vi "Read RP Modulated Configuration.vi"(8 "error in (no error)":errorcluster, 11 "Red Pitaya Modulated Digitizer in":refnum<class "Red Pitaya Modulated Digitizer.lvclass">) -> (0 "error out":errorcluster, 2 "Configuration":T1={"Pre-trigger duration"=0.01, "Post-trigger duration"=0.1, "Rate"=125000000.0, "Ranges"=[1.0], "Re-name channels"=[], "Active channels"="0:1", "External clock"=FALSE, "Modulation"={"Output delay"=0.001, "After delay"=FALSE}} {"Modulation"."Output delay" format="%#_6ps"; "Rate" format="%#_8pHz"; "Post-trigger duration" format="%#_6ps"; "Pre-trigger duration" format="%#_6ps"; "Ranges" format="%#_6pV"}, 3 "Red Pitaya Modulated Digitizer out":refnum<class "Red Pitaya Modulated Digitizer.lvclass">)   [LabVIEW 2020, in "Red Pitaya Modulated Digitizer.lvclass"]
uses:
  Red Pitaya Modulated Digitizer.lvclass
  C:/GitHub/NHMFL_Core/Libraries/Instruments/Instrument Driver/Instrument Driver.lvclass
  RP Modulated Configuration.ctl
  Modulation.ctl
  Instruments/Instrument Driver/Read User configuration.vi
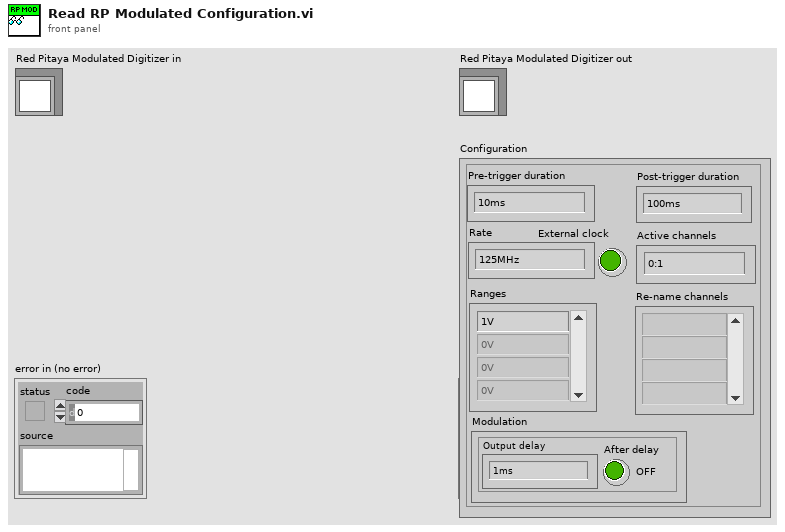
[diagram p1: front panel]
types:
  T1 = typedef "RP Modulated Configuration.ctl" = cluster{"Pre-trigger duration":dbl, "Post-trigger duration":dbl, "Rate":dbl, "Ranges":dbl[], "Re-name channels":string[], "Active channels":string, "External clock":bool, "Modulation":T2}
  T2 = typedef "Modulation.ctl" = cluster{"Output delay":dbl, "After delay":bool}
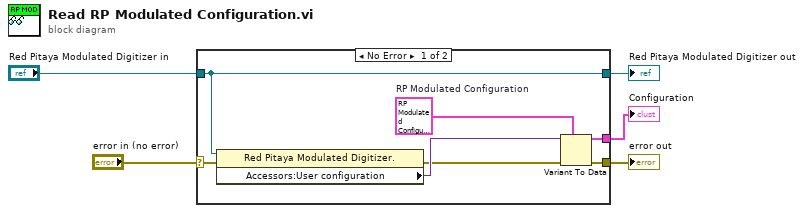
[diagram p0: block diagram]
diagram:
  n1 = case shown="No Error" "error in (no error)" {
    selector: "error in (no error)" -> [w10 w13]
    tunnel: [w8 w13] -> w4
    tunnel: [w11 w14] -> w2
    tunnel: "Red Pitaya Modulated Digitizer in" -> [w11 w14]
    tunnel: [w6 _] -> w1
    frame No Error {
      w7 = T1 {"Pre-trigger duration"=0.01, "Post-trigger duration"=0.1, "Rate"=125000000.0, "Ranges"=[1.0], "Re-name channels"=[], "Active channels"="0:1", "External clock"=FALSE, "Modulation"={"Output delay"=0.001, "After delay"=FALSE}}  # RP Modulated Configuration
      n2 = property class="Red Pitaya Modulated Digitizer."(reference=w11, error in=w10) -> (error out=w9:errorcluster, "Accessors:User configuration"=w12:variant)  [unwired: 1 out]
      n3 = Variant To Data(error in=w9, type=w7, Variant=w12) -> (data=w6:T1, error out=w8:errorcluster)
    }
    frame Error {
    }
  }
  "error out" <- w4
  "Red Pitaya Modulated Digitizer out" <- w2
  "Configuration" <- w1
